vi "Send Command.vi"(6 "Command":T1, 8 "error in":errorcluster, 10 "Value":dbl, 11 "ThorlabsLabJack in":refnum<class "ThorlabsLabJack.lvclass">) -> (0 "error out":errorcluster, 3 "ThorlabsLabJack out":refnum<class "ThorlabsLabJack.lvclass">)   [LabVIEW 2018, in "ThorlabsLabJack.lvlib" / "ThorlabsLabJack.lvclass"]
doc: "This VI will send a specific command to the Motor."
uses:
  ThorlabsLabJack.lvclass
  LWS_Base/trunk/LabVIEW/PPLs/Configuration/Axis.lvlibp/Custom Controls/Command.ctl
  LWS_Base/trunk/LabVIEW/PPLs/Configuration/Axis.lvlibp
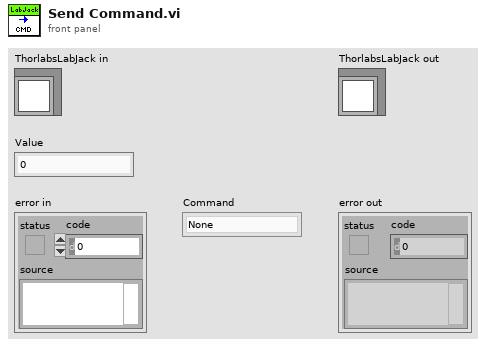
[diagram p1: front panel]
types:
  T1 = typedef "Axis.lvlibp/Command.ctl" = enum16{"None", "Home", "Renumber", "Move Absolute", "Move Relative", "Stop", "Set Run Speed", "Set Acceleration", "Set Run Current", "Set Home Offset", "Set Home Speed", "Query Current Position", "Load Defaults", "Query Status", "Lock Controls", "Unlock Controls", "Set Jog Step Size", "Set Jog Acceleration", "Set Jog Speed", "Query Homed Status", "Query Moving Status", "Reset"}
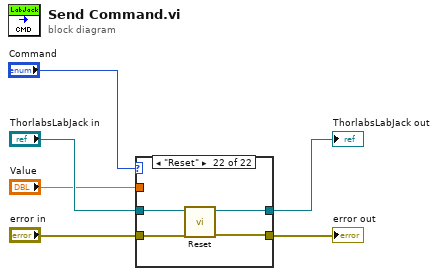
[diagram p0: block diagram]
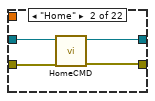
[diagram p3: hidden frame]
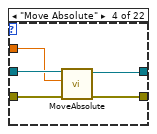
[diagram p5: hidden frame]
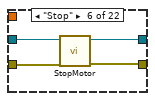
[diagram p7: hidden frame]
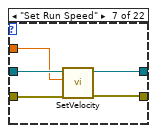
[diagram p8: hidden frame]
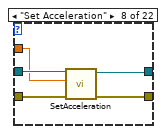
[diagram p9: hidden frame]
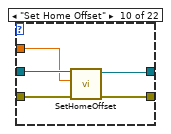
[diagram p11: hidden frame]
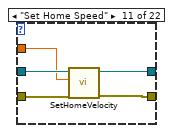
[diagram p12: hidden frame]
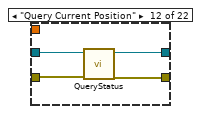
[diagram p13: hidden frame]
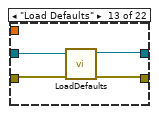
[diagram p14: hidden frame]
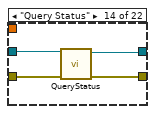
[diagram p15: hidden frame]
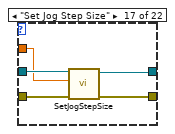
[diagram p18: hidden frame]
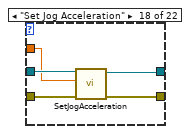
[diagram p19: hidden frame]
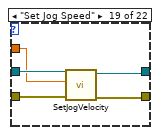
[diagram p20: hidden frame]
diagram:
  n1 = case shown="\"Reset\"" "Command" {
    tunnel: "ThorlabsLabJack in" -> [w8 w9 w14 w19 w21 w22 w30 w32 w37 w42 w47 w51 w55 w59 w61 w63 w68 w73 w78 w82 w86 w90]
    tunnel: "error in" -> [w7 w12 w13 w18 w20 w25 w27 w35 w36 w39 w44 w48 w52 w56 w60 w62 w65 w71 w76 w79 w83 w88]
    tunnel: [w8 w10 w14 w16 w21 w23 w29 w33 w37 w41 w46 w50 w54 w58 w61 w63 w67 w69 w75 w81 w85 w89] -> w3
    tunnel: [w7 w11 w13 w17 w20 w24 w26 w34 w36 w40 w45 w49 w53 w57 w60 w62 w64 w70 w74 w80 w84 w87] -> w2
    tunnel: "Value" -> [_ _ _ w15 _ _ w28 w31 _ w38 w43 _ _ _ _ _ w66 w72 w77 _ _ _]
    frame "None", Default {
    }
    frame "Home" {
      n2 = call "HomeCMD.vi"("error in (no error)"=w12, "ThorlabsLabJack in"=w9) -> ("error out"=w11:errorcluster, "ThorlabsLabJack out"=w10:refnum<class "ThorlabsLabJack.lvclass">)  [unwired: 8 in]
    }
    frame "Renumber" {
    }
    frame "Move Absolute" {
      n3 = call "MoveAbsolute.vi"("error in (no error)"=w18, "Move Abs Value"=w15, "ThorlabsLabJack in"=w19) -> ("error out"=w17:errorcluster, "ThorlabsLabJack out"=w16:refnum<class "ThorlabsLabJack.lvclass">)  [unwired: 7 in]
    }
    frame "Move Relative" {
    }
    frame "Stop" {
      n4 = call "StopMotor.vi"("error in (no error)"=w25, "ThorlabsLabJack in"=w22) -> ("error out"=w24:errorcluster, "ThorlabsLabJack out"=w23:refnum<class "ThorlabsLabJack.lvclass">)  [unwired: 8 in]
    }
    frame "Set Run Speed" {
      n5 = call "SetVelocity.vi"("error in (no error)"=w27, "Velocity"=w28, "ThorlabsLabJack in"=w30) -> ("error out"=w26:errorcluster, "ThorlabsLabJack out"=w29:refnum<class "ThorlabsLabJack.lvclass">)  [unwired: 7 in]
    }
    frame "Set Acceleration" {
      n6 = call "SetAcceleration.vi"("error in (no error)"=w35, "Acceleration"=w31, "ThorlabsLabJack in"=w32) -> ("error out"=w34:errorcluster, "ThorlabsLabJack out"=w33:refnum<class "ThorlabsLabJack.lvclass">)  [unwired: 7 in]
    }
    frame "Set Run Current" {
    }
    frame "Set Home Offset" {
      n7 = call "SetHomeOffset.vi"("error in (no error)"=w39, "Offset"=w38, "ThorlabsLabJack in"=w42) -> ("error out"=w40:errorcluster, "ThorlabsLabJack out"=w41:refnum<class "ThorlabsLabJack.lvclass">)  [unwired: 7 in]
    }
    frame "Set Home Speed" {
      n8 = call "SetHomeVelocity.vi"("error in (no error)"=w44, "Velocity"=w43, "ThorlabsLabJack in"=w47) -> ("error out"=w45:errorcluster, "ThorlabsLabJack out"=w46:refnum<class "ThorlabsLabJack.lvclass">)  [unwired: 7 in]
    }
    frame "Query Current Position" {
      n9 = call "QueryStatus.vi"("error in (no error)"=w48, "ThorlabsLabJack in"=w51) -> ("error out"=w49:errorcluster, "ThorlabsLabJack out"=w50:refnum<class "ThorlabsLabJack.lvclass">)  [unwired: 8 in]
    }
    frame "Load Defaults" {
      n10 = call "LoadDefaults.vi"("error in (no error)"=w52, "ThorlabsLabJack in"=w55) -> ("error out"=w53:errorcluster, "ThorlabsLabJack out"=w54:refnum<class "ThorlabsLabJack.lvclass">)  [unwired: 8 in]
    }
    frame "Query Status" {
      n11 = call "QueryStatus.vi"("error in (no error)"=w56, "ThorlabsLabJack in"=w59) -> ("error out"=w57:errorcluster, "ThorlabsLabJack out"=w58:refnum<class "ThorlabsLabJack.lvclass">)  [unwired: 8 in]
    }
    frame "Lock Controls" {
    }
    frame "Unlock Controls" {
    }
    frame "Set Jog Step Size" {
      n12 = call "SetJogStepSize.vi"("error in (no error)"=w65, "Jog Step Size"=w66, "ThorlabsLabJack in"=w68) -> ("error out"=w64:errorcluster, "ThorlabsLabJack out"=w67:refnum<class "ThorlabsLabJack.lvclass">)  [unwired: 7 in]
    }
    frame "Set Jog Acceleration" {
      n13 = call "SetJogAcceleration.vi"("error in (no error)"=w71, "Jog Acceleration"=w72, "ThorlabsLabJack in"=w73) -> ("error out"=w70:errorcluster, "ThorlabsLabJack out"=w69:refnum<class "ThorlabsLabJack.lvclass">)  [unwired: 7 in]
    }
    frame "Set Jog Speed" {
      n14 = call "SetJogVelocity.vi"("error in (no error)"=w76, "Jog Velocity"=w77, "ThorlabsLabJack in"=w78) -> ("error out"=w74:errorcluster, "ThorlabsLabJack out"=w75:refnum<class "ThorlabsLabJack.lvclass">)  [unwired: 7 in]
    }
    frame "Query Homed Status" {
      n15 = call "QueryStatus.vi"("error in (no error)"=w79, "ThorlabsLabJack in"=w82) -> ("error out"=w80:errorcluster, "ThorlabsLabJack out"=w81:refnum<class "ThorlabsLabJack.lvclass">)  [unwired: 8 in]
    }
    frame "Query Moving Status" {
      n16 = call "QueryStatus.vi"("error in (no error)"=w83, "ThorlabsLabJack in"=w86) -> ("error out"=w84:errorcluster, "ThorlabsLabJack out"=w85:refnum<class "ThorlabsLabJack.lvclass">)  [unwired: 8 in]
    }
    frame "Reset" {
      n17 = call "Reset.vi"("error in (no error)"=w88, "ThorlabsLabJack in"=w90) -> ("error out"=w87:errorcluster, "ThorlabsLabJack out"=w89:refnum<class "ThorlabsLabJack.lvclass">)  [unwired: 8 in]
    }
  }
  "error out" <- w2
  "ThorlabsLabJack out" <- w3
